vi "S7COMM - Parse Response - Evaluate Header.vi"(7 "S7":refnum<class "S7NetCom.lvclass">, 8 "error in (no error)":errorcluster, 11 "S7 PDU Data in":T1 format="0x%02x") -> (0 "error out":errorcluster, 2 "Sequence Number":u16, 3 "S7COMM Param and Data":T1 format="0x%02x", 5 "S7 out":refnum<class "S7NetCom.lvclass">)   [LabVIEW 2014, in "S7NetCom.lvclass"]
uses:
  S7NetCom.lvclass
  Controls/S7NetCom_HexByteArray.ctl
  Controls/S7NetCom_HexByte.ctl
  S7NetCom.lvclass/S7NetCom.ctl
  S7COMM - Response Protocol Header Mismatch-error.vi
  S7COMM - Response Message Type Mismatch-error.vi
  S7COMM - Response Sequence Number Mismatch-error.vi
panel:
  out "Parameter Length":u16
  out "Data Length":u16
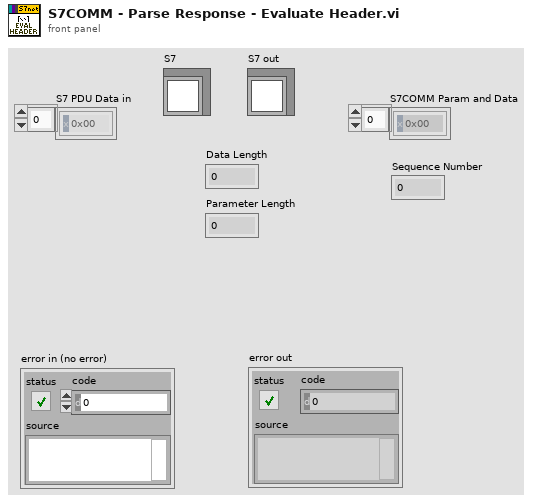
[diagram p1: front panel]
types:
  T1 = typedef "S7NetCom.lvclass/S7NetCom_HexByteArray.ctl" = T2[]
  T2 = typedef "S7NetCom.lvclass/S7NetCom_HexByte.ctl" = u8
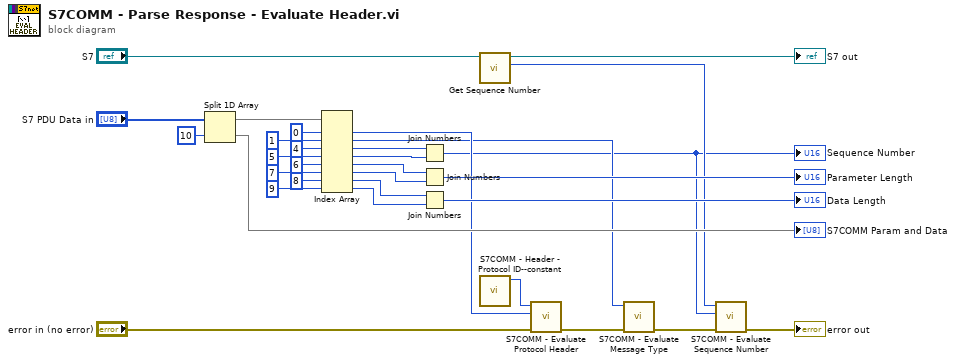
[diagram p0: block diagram]
diagram:
  n1 = Split 1D Array(array="S7 PDU Data in", index=10) -> (first subarray=w13:T1, second subarray=→"S7COMM Param and Data":T1)
  n2 = Index Array(array=w13, index #1=0, index #2=1, index #3=4, index #4=5, index #5=6, index #6=7, index #7=8, index #8=9) -> (element #1=w5:T2, element #2=w3:T2, element #3=w26:T2, element #4=w27:T2, element #5=w28:T2, element #6=w29:T2, element #7=w30:T2, element #8=w31:T2)
  n3 = Join Numbers(hi=w26, lo=w27) -> ((hi.lo)=w1:u16)
  "Sequence Number" <- w1
  n4 = Join Numbers(hi=w28, lo=w29) -> ((hi.lo)=→"Parameter Length":u16)
  n5 = Join Numbers(hi=w30, lo=w31) -> ((hi.lo)=→"Data Length":u16)
  n6 = call "Get Sequence Number.vi"("S7NetCom in"="S7") -> ("Sequence No."=w2:u16, "S7NetCom out"=→"S7 out":refnum<class "S7NetCom.lvclass">)  [unwired: 9 in]
  n7 = call "S7COMM - Header - Protocol ID--constant.vi"() -> ("Protocol ID"=w4:u8)  [unwired: 11 in]
  n8 = call "S7COMM - Evaluate Protocol Header.vi"("error in (no error)"="error in (no error)", "PLC Response Value"=w5, "S7 Protocol ID"=w4) -> ("error out"=w8:errorcluster)  [unwired: 8 in]
  n9 = call "S7COMM - Evaluate Message Type.vi"("error in (no error)"=w8, "PLC Message Type"=w3) -> ("error out"=w7:errorcluster)  [unwired: 9 in]
  n10 = call "S7COMM - Evaluate Sequence Number.vi"("error in (no error)"=w7, "PLC Response Seq No"=w1, "Sent Seq No."=w2) -> ("error out"=→"error out":errorcluster)  [unwired: 8 in]
